vi "bigmcs.vi"(5 "Spinal Column Out":T2={"Red MOT 88 Inputs"={"Active Device"="", "Active Channels"=[], "Waveform Parameters"=[], "Active Phases"=[], "Phase Times"=[], "Trigger Channel"=""}, "6713 Blue MOT"={"Active Device"="", "Active Channels"=[], "Waveform Parameters"=[], "Active Phases"=[], "Phase Times"=[], "Trigger Channel"="", "FIFO Buffer Size"=0.0}, "Instructions"=[], "Red MOT 87 Inputs"={"Active Device"="", "Active Channels"=[], "Waveform Parameters"=[], "Active Phases"=[], "Phase Times"=[], "Trigger Channel"=""}, "ODT Params"={"Waveform Parameters"=[], "Active Phases"=[], "Active Channels"=[], "Phase Times (s)"=[], "Active Device"="", "Trigger Channel"="", "Evaporation Phase"=0.0, "Evaporation Channel"=0.0}, "Agilent E3631A Settings"={"VISA resource name"="", "Voltage Set (6V max)"=0.0, "Current Set (5A max)"=0.0, "Voltage Set (25V max)"=0.0, "Current Set (1A max)"=0.0}, "PixelFly Initialization"={"Exposure mode"=0, "exp time"=0, "exp level"=0, "gain"=0, "boardid in"=0, "offset"=0, "V bin"=0, "H bin"=0, "trigger"=FALSE, "Bit depth"=0}, "Scan Parameters"={"Initial Values"=[], "Final Values"=[], "Step Sizes"=[], "Parameters to Change"=[], "Channels to Change"=[], "Number of Parameters to Scan"=0, "Parameter Nickname (no spaces)"=[], "Scan Base Name"="", "Raw_Data Folder"=path "", "ROI Parameters"={"Background Radius"=0.0, "Atom Radius"=0.0, "X Center"=0.0, "Y Center"=0.0}, "Drop Time (ms)"=0.0, "ODT VCA 1 Channel"=0.0, "ODT VCA 2 Channel"=0.0, "Phases To Change"=[], "Scan Pulseblaster Channel With Parameter"={"Change PB Time Toggle"=FALSE, "PB Channel"=0.0, "Parameter Number"=0.0}, "Preserve Waveform\nContinuity"=FALSE, "Generated Array Type"=enum."Custom Array From File", "Principle Quantum #"=0, "Angular Momentum"=enum."s", "Ramp Delay Channel"=0, "ODT Hold Channel"=0, "MCS ROI Min"=0, "MCS ROI Max"=0, "Master Batch Fourth Column"=0.0}, "MCS Parameters"={"Scan Length (Bins)"=0.0, "Dwell Time (s)"=0.0, "Gate Channel Settings"={"Threshold (V)"=0.0, "Edge"=enum."Falling", "Input Impedence"=enum."1k Ohm"}, "Trig Channel Settings"={"Threshold (V)"=0.0, "Edge"=enum."Falling", "Input Impedence"=enum."1k Ohm"}, "Input 1 Settings"={"Threshold (V)"=0.0, "Edge"=enum."Falling", "Input Impedence"=enum."1k Ohm"}, "Input 2 Settings"={"Threshold (V)"=0.0, "Edge"=enum."Falling", "Input Impedence"=enum."1k Ohm"}, "Number of Sweeps"=0, "Number of Sequential Cycles"=0.0, "Number of Sequences"=0.0, "Sweep Preset"=FALSE, "Sequential Mode"=FALSE, "DAC 1 Ramp Settings"={"Ramp Mode"=enum."Fixed", "Ramp Start Value (V)"=0.0, "Ramp Length (Steps)"=0, "Step Width (bins)"=0, "Step Size (V)"=0.0}, "DAC 2 Output (V)"=0.0, "SYNC Output"=enum."40 MHz Clock", "ROI Min"=0, "ROI Max"=0, "Dual MCS Mode"=FALSE, "DAC 2 Toggle"=FALSE, "MCS on/off"=FALSE, "ROI Max 2"=1, "ROI Min 2"=0, "Sum ROI Only"=FALSE, "Use ROI For \nEach Loop"=FALSE}, "PicoScope"={"Channel A Settings"={"Enabled"=FALSE, "Coupling"=0, "Range"=0, "Analogue Offset"=0.0}, "Channel B Settings"={"Enabled"=FALSE, "Coupling"=0, "Range"=0, "Analogue Offset"=0.0}, "Trigger Options"={"Trigger Enabled"=FALSE, "Trigger Source"=enum."Channel A", "Trigger Threshold (-5 to 5 V)"=0.0, "Trigger Slope"=0, "Trigger Delay (ms)"=0.0, "Auto Trigger Time (ms)"=0}, "Pico Scope Inititalization Settings"={"USB Power"=FALSE, "Use Serial Number"=FALSE, "Resolution"=0, "Serial Number"="", "Handle"=0}, "Use PicoScope?"=FALSE, "Acquisition Settings"={"Pre Trigger Time (s)"=0.0, "Post Trigger Time (s)"=0.0, "Resolution (s)"=0.0, "Four Channel Device"=FALSE, "Number of Captures"=0.0}}, "Ramp Delay Settings"={"Insert Delays"=FALSE, "Number of loops"=0, "Insert after instruction"=0, "Random"=FALSE, "Initial Delay Time (s)"=0.0, "Final Delay Time (s)"=0.0, "Delay Step (s)"=0.0, "Delay Column"=0.0, "Loop Hold Column"=0.0, "Field Ramp Column"=0.0, "Excitation Column"=0.0, "Hold + Delay + Excitation Time"=0.0, "Ascending/Descending"=FALSE, "Subroutine A"=[]}, "6229 Green Lattice Inputs"={"Active Device"="", "Active Channels"=[], "Waveform Parameters"=[], "Active Phases"=[], "Phase Times"=[], "Trigger Channel"="", "FIFO Buffer Size"=0.0}, "Synth Controls 1"={"Channel Settings"=[], "Active Channels"=[], "COM Port"="", "Table Mode"={"Table Mode On/Off"=FALSE, "Initial Frequency (MHz)"=0.0, "FinalFreq"=0.0, "Frequency Step (MHz)"=0.0, "Ascending/Descending"=FALSE, "Random"=FALSE}}, "Synth Controls 2"={"Channel Settings"=[], "Active Channels"=[], "COM Port"="", "Table Mode"={"Table Mode On/Off"=FALSE, "Initial Frequency (MHz)"=0.0, "FinalFreq"=0.0, "Frequency Step (MHz)"=0.0, "Ascending/Descending"=FALSE, "Random"=FALSE}}, "Indicator References"={"Blue MOT Waveform Graph"=refnum, "Red 88 Waveform Graph"=refnum, "Red 87 Waveform Graph"=refnum, "ODT Waveform Graph"=refnum, "Green Lattice Waveform Graph"=refnum, "Agilent E3631A Measurements"=refnum}} {"Red MOT 88 Inputs"."Phase Times" format="%.0p"; "Red MOT 88 Inputs"."Waveform Parameters"."Degree" min=1; "6713 Blue MOT"."Phase Times" format="%.3f"; "Instructions"."Time (s)" min=5e-08 format="%.2p"; "Instructions"."Op Code" items=["Continue", "Stop", "Loop", "End Loop", "JSR", "RTS", "Go To", "Long Delay", "Wait"]; "Instructions"."Instruct Data" format="%#.2p"; "Red MOT 87 Inputs"."Phase Times" format="%.0p"; "Red MOT 87 Inputs"."Waveform Parameters"."Degree" min=1; "ODT Params"."Evaporation Channel" min=0.0 max=1.0 step=1.0; "ODT Params"."Evaporation Phase" min=0.0 max=4.0 step=1.0; "ODT Params"."Phase Times (s)" format="%#_6p"; "Agilent E3631A Settings"."Current Set (1A max)" format="%.3g"; "Agilent E3631A Settings"."Voltage Set (25V max)" format="%.3g"; "Agilent E3631A Settings"."Current Set (5A max)" format="%.3g"; "Agilent E3631A Settings"."Voltage Set (6V max)" format="%.3g"; "PixelFly Initialization"."Bit depth" items=["2"=1]; "PixelFly Initialization"."H bin" items=["1", "2"]; "PixelFly Initialization"."V bin" items=["1", "2"]; "PixelFly Initialization"."boardid in" min=0 max=3 step=1; "PixelFly Initialization"."gain" items=["Low (X1)", "High (X2)"]; "PixelFly Initialization"."exp level" min=0 max=255 step=1; "PixelFly Initialization"."exp time" min=1 max=10000; "PixelFly Initialization"."Exposure mode" items=["Asynch shutter", "Double shot", "Video mode", "Auto exposure"]; "Scan Parameters"."Drop Time (ms)" min=1.0; "Scan Parameters"."Number of Parameters to Scan" min=1; "MCS Parameters"."ROI Max 2" min=1; "MCS Parameters"."ROI Min 2" min=0; "MCS Parameters"."ROI Max" min=1; "MCS Parameters"."ROI Min" min=0; "MCS Parameters"."DAC 2 Output (V)" min=-10.0 max=10.0 step=0.00488; "MCS Parameters"."DAC 1 Ramp Settings"."Step Size (V)" min=0.0 max=10.0 step=0.00244 format="%#_4g"; "MCS Parameters"."DAC 1 Ramp Settings"."Step Width (bins)" min=1; "MCS Parameters"."DAC 1 Ramp Settings"."Ramp Length (Steps)" min=1; "MCS Parameters"."DAC 1 Ramp Settings"."Ramp Start Value (V)" min=0.0 max=10.0 step=0.00244; "MCS Parameters"."Number of Sweeps" min=0 format="%.0p"; "MCS Parameters"."Input 2 Settings"."Threshold (V)" min=-2.5 max=2.5 step=0.001; "MCS Parameters"."Input 1 Settings"."Threshold (V)" min=-2.5 max=2.5 step=0.001; "MCS Parameters"."Trig Channel Settings"."Threshold (V)" min=-2.5 max=2.5 step=0.001; "MCS Parameters"."Gate Channel Settings"."Threshold (V)" min=-2.5 max=2.5 step=0.001; "MCS Parameters"."Dwell Time (s)" min=1e-07 step=2.5e-08 format="%#_6p"; "MCS Parameters"."Scan Length (Bins)" min=64.0 max=524288.0 format="%#_7f"; "PicoScope"."Acquisition Settings"."Resolution (s)" min=8e-09 max=34.36 step=8e-09 format="%#_6p"; "PicoScope"."Acquisition Settings"."Post Trigger Time (s)" min=0.0 format="%#_6p"; "PicoScope"."Acquisition Settings"."Pre Trigger Time (s)" min=0.0 format="%#_6p"; "PicoScope"."Pico Scope Inititalization Settings"."Resolution" items=["8-bit", "12-bit", "14-bit", "15-bit (max. 2 ch.)", "16-bit (max. 1 ch.)"]; "PicoScope"."Trigger Options"."Trigger Slope" items=["Rising"=2, "Falling"=3]; "PicoScope"."Channel B Settings"."Range" items=["10 mV", "20 mV", "50 mV", "100 mV", "200 mV", "500 mV", "1 V", "2 V", "5 V", "10 V", "20 V", "50 V ", "100 V"]; "PicoScope"."Channel B Settings"."Coupling" items=["AC", "DC"]; "PicoScope"."Channel A Settings"."Range" items=["10 mV", "20 mV", "50 mV", "100 mV", "200 mV", "500 mV", "1 V", "2 V", "5 V", "10 V", "20 V", "50 V ", "100 V"]; "PicoScope"."Channel A Settings"."Coupling" items=["AC", "DC"]; "Ramp Delay Settings"."Subroutine A"."Time (s)" min=5e-08 format="%.2p"; "Ramp Delay Settings"."Subroutine A"."Op Code" items=["Continue", "Stop", "Loop", "End Loop", "JSR", "RTS", "Go To", "Long Delay", "Wait"]; "Ramp Delay Settings"."Subroutine A"."Instruct Data" format="%#.2p"; "Ramp Delay Settings"."Insert after instruction" min=0; "Ramp Delay Settings"."Delay Step (s)" min=5e-08 format="%#_6p"; "Ramp Delay Settings"."Final Delay Time (s)" min=5e-08 format="%#_6p"; "Ramp Delay Settings"."Initial Delay Time (s)" min=5e-08 format="%#_6p"; "6229 Green Lattice Inputs"."Phase Times" format="%.3f"; "6229 Green Lattice Inputs"."Waveform Parameters"."Degree" min=1}, 7 "Synth Freq":dbl, 8 "MCS Counts Out":u32[][](graph)=[[0, 0, 0, 0, 0, 0, 0, 0, 0, 0, 0, 0, 0, 0, 0, 0, 0, 0, 0, 0, 0, 0, 0, 0, 0, 0, 0, 0, 0, 0, 0, 0, 0, 0, 0, 0, 0, 0, 0, 0, 0, 0, 0, 0, 0, 0, 0, 0, 0, 0, 0, 0, 0, 0, 0, 0, 0, 0, 0, 0, 0, 0, 0, 0, 0, 0, 0, 0, 0, 0, 0, 0, 0, 1, 1, 0, 0, 0, 0, 0, 2, 0, 0, 0, 0, 0, 0, 0, 0, 0, 0, 0, 0, 1, 3, 1, 0, 0, 0, 0, 0, 0, 0, 0, 0, 0, 0, 0, 0, 0, 0, 0, 0, 0, 0, 0, 0, 0, 0, 0, 0, 0, 0, 0, 0, 0, 0, 0, 0, 0, 0, 0, 0, 0, 0, 0, 0, 0, 0, 0, 0, 0, 0, 0, 0, 0, 0, 0, 0, 0, 0, 0, 0, 0, 0, 0, 0, 0, 0, 0, 0, 0, 0, 0, 0, 0, 0, 0, 0, 0, 0, 0, 0, 0, 1, 0, 0, 0, 0, 0, 0, 0, 0, 0, 0, 0, 0, 0, 0, 0, 0, 0, 0, 0, 0, 0, 0, 0, 0, 0, 0, 0, 0, 0, 0, 0, 0, 0, 0, 0, 0, 0, 0, 0, 0, 0, 0, 0, 0, 0, 0, 0, 0, 0, 0, 0, 0, 0, 0, 0, 0, 0, 0, 0, 0, 0, 0, 0, 0, 0, 0, 0, 0, 0, 0, 0, 0, 0, 0, 0]], 9 "Tau Array":dbl[](array[numeric]), 10 "Sum #":dbl, 11 "Sum in":u32[][](graph)) -> ()   [LabVIEW 2015]
uses:
  Controls/Spinal Column/spinal_column.ctl
  6733_Red_MOT/6733_control_panel.ctl
  6733_Red_MOT/6733_waveform_parameter_array.ctl
  6733_Red_MOT/6733_waveform_item.ctl
  6733_Red_MOT/Neutral_voltage_conversion_control.ctl
  Controls/6713/6713_waveform_generation.ctl
  Controls/6713/6713_waveform_parameter_array.ctl
  Controls/6713/6713_static_waveform_item.ctl
  Controls/PulseBlaster/Instructions_Cluster.ctl
  Neutral_DAQ/6221 arb waveforms/6221_panel.ctl
  Neutral_DAQ/6221 arb waveforms/6221_waveform_param.ctl
  Controls/Agilent E3631A/Settings_Control.ctl
  Controls/PixelFly/Camera_Initialization.ctl
  Controls/ScanParameters/ScanParametersPanel.ctl
  Controls/ScanParameters/ParameterToChange.ctl
  Controls/ScanParameters/ROI_set.ctl
  Controls/ScanParameters/ScanPBandParam.ctl
  Controls/MCS/mcs_control_panel.ctl
  Controls/MCS/mcs_channel.ctl
  Controls/MCS/ramp_control.ctl
  Controls/PicoScope/pico_control_panel.ctl
  Controls/PicoScope/pico_channel_settings.ctl
  Controls/PicoScope/pico_trigger.ctl
  Controls/PicoScope/pico_init_settings.ctl
  Controls/PulseBlaster/delay_control_3..ctl
  Controls/6229/6229_arb_waveform_generation.ctl
  Controls/Synth_409b/Synth_controls.ctl
  Controls/Synth_409b/synth_channel.ctl
  Controls/Synth_409b/table_mode.ctl
  <vilib>/Utility/file.llb/Write To Spreadsheet File (DBL).vi
  <vilib>/Analysis/NI_AALPro.lvlib
panel:
  in  "Trace Scale":bool caption="Linear / Logrithmic"
  in  "Sum Scale":bool caption="Linear / Logrithmic"
  in  "Record Lifetime":bool
  in  "file path (dialog if empty)":path
  out "Lifetime Running Average":dbl[][](graph)
  out "Sum graph":u32[][](graph)
  out "error out":errorcluster
  out "XY Graph 3":cluster{"Tau Array":dbl[], u32[]}[](graph)
  out "Lifetimes":dbl[][](graph)
  out "Lifetimes":dbl[](array[numeric])
  in  "parameter bounds":T1={"amp min"=-inf, "amp max"=inf, "damping min"=-inf, "damping max"=inf, "offset min"=0.0, "offset max"=0.0}
  in  "Clear Graph":bool
  out "appended array":cluster{"Sum #":dbl, "Synth Freq":dbl}[](array[cluster])
  out "XY Graph":cluster{"X":dbl, "Y":dbl}[](graph)
  # "Channel 0"
  # "Channel 1"
  # "Channel 2"
  # "Channel 3"
  # "Channel 4"
  # "Channel 5"
  # "Channel 7"
  # "Channel 7"
  # "(0) 689 Center Freq"
  # "(1) 689 Dither Amp"
  # "(2) 689 Power Lock"
  # "(3) Red MOT Field Grad"
  # "Channel 0"
  # "Channel 1"
  # "Channel 2"
  # "Channel 3"
  # "Channel 4"
  # "Channel 5"
  # "Channel 7"
  # "Channel 7"
  # "6V Output Settings"
  # "25V Output Settings"
  # "Select a PB Channel to set with a phase time\nfor evaporation or whatever"
  # "(0) Arm A"
  # "(1) Arm B"
  # "(2) Arm C"
  # "(3) Unused"
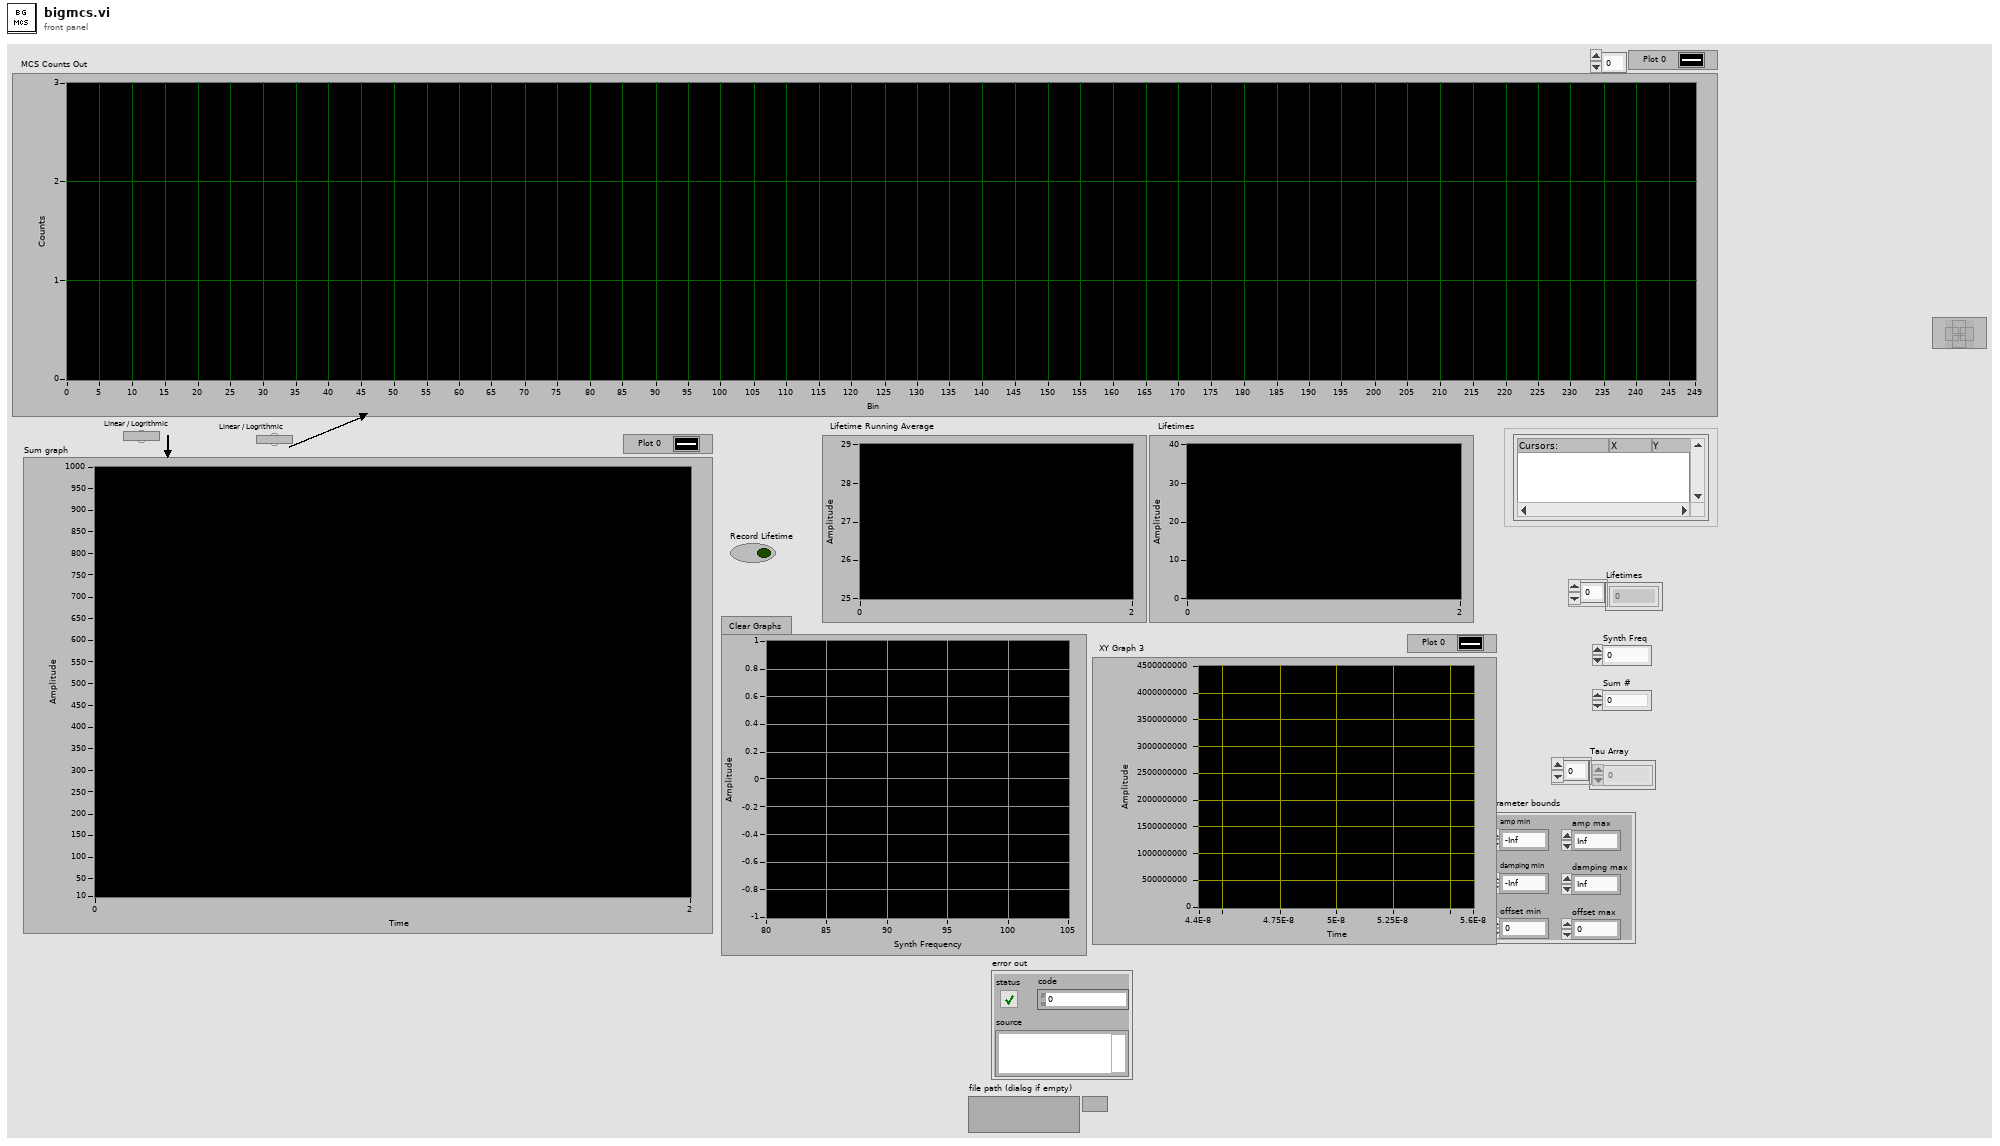
[diagram p1: front panel]
types:
  T1 = cluster{"amp min":dbl, "amp max":dbl, "damping min":dbl, "damping max":dbl, "offset min":dbl, "offset max":dbl}
  T2 = typedef "spinal_column.ctl" = cluster{"Red MOT 88 Inputs":T3, "6713 Blue MOT":T7, "Instructions":T10, "Red MOT 87 Inputs":T3, "ODT Params":T11, "Agilent E3631A Settings":T13, "PixelFly Initialization":T14, "Scan Parameters":T15, "MCS Parameters":T19, "PicoScope":T22, "Ramp Delay Settings":T26, "6229 Green Lattice Inputs":T27, "Synth Controls 1":T28, "Synth Controls 2":T28, "Indicator References":cluster{"Blue MOT Waveform Graph":refnum<vi>, "Red 88 Waveform Graph":refnum<vi>, "Red 87 Waveform Graph":refnum<vi>, "ODT Waveform Graph":refnum<vi>, "Green Lattice Waveform Graph":refnum<vi>, "Agilent E3631A Measurements":refnum<vi>}}
  T3 = typedef "6733_control_panel.ctl" = cluster{"Active Device":string, "Active Channels":bool[], "Waveform Parameters":T4, "Active Phases":bool[], "Phase Times":dbl[], "Trigger Channel":tag}
  T4 = typedef "6733_waveform_parameter_array.ctl" = T5[][]
  T5 = typedef "6733_waveform_item.ctl" = cluster{"Function":enum16{"Polynomial", "Exponential", "Constant"}, "Initial":dbl, "Final":dbl, "Degree":i8, "Nickname":string, "Conversion":T6, "Constant":dbl}
  T6 = typedef "Neutral_voltage_conversion_control.ctl" = enum16{"Volts", "B Field Grad (G/cm)", "Red MOT Center Freq (MHz)", "Red Dither Pk(kHz)", "Red Power (mW)", "ODT Sheet Trap Power (W)", "ODT Loading Trap Power (W)"}
  T7 = typedef "6713_waveform_generation.ctl" = cluster{"Active Device":string, "Active Channels":bool[], "Waveform Parameters":T8, "Active Phases":bool[], "Phase Times":dbl[], "Trigger Channel":tag, "FIFO Buffer Size":dbl}
  T8 = typedef "6713_waveform_parameter_array.ctl" = T9[][]
  T9 = typedef "6713_static_waveform_item.ctl" = cluster{"Constant":dbl, "Nickname":string, "Conversion":T6}
  T10 = typedef "Instructions_Cluster.ctl" = cluster{"Instruct Data":i32, "Op Code":i32, "Flags":bool[], "Comments":string, "Time (s)":dbl, "Column Number":string, "Array":string[]}[]
  T11 = typedef "6221_panel.ctl" = cluster{"Waveform Parameters":T12[][], "Active Phases":bool[], "Active Channels":bool[], "Phase Times (s)":dbl[], "Active Device":string, "Trigger Channel":tag, "Evaporation Phase":dbl, "Evaporation Channel":dbl}
  T12 = typedef "6221_waveform_param.ctl" = cluster{"Initial Value":dbl, "Final Value":dbl, "Tau":dbl, "Eta":dbl, "Nickname":string, "Enum":enum16{"Volts to Volts", "Power Law", "Evaporation Formula"}, "Conversion":T6}
  T13 = typedef "Settings_Control.ctl" = cluster{"VISA resource name":refnum<visa-resource-name>, "Voltage Set (6V max)":dbl, "Current Set (5A max)":dbl, "Voltage Set (25V max)":dbl, "Current Set (1A max)":dbl}
  T14 = typedef "Camera_Initialization.ctl" = cluster{"Exposure mode":u16, "exp time":i32, "exp level":i32, "gain":i32, "boardid in":i32, "offset":i32, "V bin":i32, "H bin":i32, "trigger":bool, "Bit depth":i32}
  T15 = typedef "ScanParametersPanel.ctl" = cluster{"Initial Values":dbl[], "Final Values":dbl[], "Step Sizes":dbl[], "Parameters to Change":T16[], "Channels to Change":dbl[], "Number of Parameters to Scan":i32, "Parameter Nickname (no spaces)":string[], "Scan Base Name":string, "Raw_Data Folder":path, "ROI Parameters":T17, "Drop Time (ms)":dbl, "ODT VCA 1 Channel":dbl, "ODT VCA 2 Channel":dbl, "Phases To Change":dbl[], "Scan Pulseblaster Channel With Parameter":T18, "Preserve Waveform\nContinuity":bool, "Generated Array Type":enum16{"Custom Array From File", "Default (old way)"}, "Principle Quantum #":i32, "Angular Momentum":enum16{"s", "p", "d", "f", "g", "h"}, "Ramp Delay Channel":i32, "ODT Hold Channel":i32, "MCS ROI Min":i32, "MCS ROI Max":i32, "Master Batch Fourth Column":dbl}
  T16 = typedef "ParameterToChange.ctl" = enum16{"Delay single delay time", "Dummy Variable", "Delay Exposure", "PB Loops", "Number of Delay Loops", "Subroutine A Time", "Subroutine B Time", "Synth Amplitude", "Synth Frequency", "Synth Phase", "ODT Params Phase Time", "ODT Params Tau", "ODT Params Final Voltage", "ODT Params Initial Voltage", "ODT Params Eta", "Red Mot 88 Phase Time", "Red Mot 87 Phase Time", "Red Mot 88 Final Voltage", "Red Mot 88 Initial Voltage", "Red Mot 87 Final Voltage", "Red Mot 87 Initial Voltage", "PulseBlaster", "6713 Voltage"}
  T17 = typedef "ROI_set.ctl" = cluster{"Background Radius":dbl, "Atom Radius":dbl, "X Center":dbl, "Y Center":dbl}
  T18 = typedef "ScanPBandParam.ctl" = cluster{"Change PB Time Toggle":bool, "PB Channel":dbl, "Parameter Number":dbl}
  T19 = typedef "mcs_control_panel.ctl" = cluster{"Scan Length (Bins)":dbl, "Dwell Time (s)":dbl, "Gate Channel Settings":T20, "Trig Channel Settings":T20, "Input 1 Settings":T20, "Input 2 Settings":T20, "Number of Sweeps":i32, "Number of Sequential Cycles":dbl, "Number of Sequences":dbl, "Sweep Preset":bool, "Sequential Mode":bool, "DAC 1 Ramp Settings":T21, "DAC 2 Output (V)":dbl, "SYNC Output":enum16{"40 MHz Clock", "Gate Disc Signal", "Trigger Disc Signal", "Counter 1 Disc Signal", "Counter 2 Disc Signal", "Definitely Not Used", "Not Used", "1 kHz Signal", "Also Not Used", "MCS On/Off", "End of Time Bin", "Ramp Increment Trig", "Step Count Trigger", "'GO'-Line", "Ramp Down Trigger", "Logic 1"}, "ROI Min":i32, "ROI Max":i32, "Dual MCS Mode":bool, "DAC 2 Toggle":bool, "MCS on/off":bool, "ROI Max 2":i32, "ROI Min 2":i32, "Sum ROI Only":bool, "Use ROI For \nEach Loop":bool}
  T20 = typedef "mcs_channel.ctl" = cluster{"Threshold (V)":dbl, "Edge":enum16{"Falling", "Rising"}, "Input Impedence":enum16{"1k Ohm", "50 Ohm"}}
  T21 = typedef "ramp_control.ctl" = cluster{"Ramp Mode":enum16{"Fixed", "Triangle", "Sawtooth"}, "Ramp Start Value (V)":dbl, "Ramp Length (Steps)":i32, "Step Width (bins)":i32, "Step Size (V)":dbl}
  T22 = typedef "pico_control_panel.ctl" = cluster{"Channel A Settings":T23, "Channel B Settings":T23, "Trigger Options":T24, "Pico Scope Inititalization Settings":T25, "Use PicoScope?":bool, "Acquisition Settings":cluster{"Pre Trigger Time (s)":dbl, "Post Trigger Time (s)":dbl, "Resolution (s)":dbl, "Four Channel Device":bool, "Number of Captures":dbl}}
  T23 = typedef "pico_channel_settings.ctl" = cluster{"Enabled":bool, "Coupling":i16, "Range":u16, "Analogue Offset":sgl}
  T24 = typedef "pico_trigger.ctl" = cluster{"Trigger Enabled":bool, "Trigger Source":enum16{"Channel A", "Channel B", "Channel C", "Channel D", "Ext."}, "Trigger Threshold (-5 to 5 V)":dbl, "Trigger Slope":u16, "Trigger Delay (ms)":dbl, "Auto Trigger Time (ms)":i16}
  T25 = typedef "pico_init_settings.ctl" = cluster{"USB Power":bool, "Use Serial Number":bool, "Resolution":i32, "Serial Number":string, "Handle":i16}
  T26 = typedef "delay_control_3..ctl" = cluster{"Insert Delays":bool, "Number of loops":i32, "Insert after instruction":i32, "Random":bool, "Initial Delay Time (s)":dbl, "Final Delay Time (s)":dbl, "Delay Step (s)":dbl, "Delay Column":dbl, "Loop Hold Column":dbl, "Field Ramp Column":dbl, "Excitation Column":dbl, "Hold + Delay + Excitation Time":dbl, "Ascending/Descending":bool, "Subroutine A":T10}
  T27 = typedef "6229_arb_waveform_generation.ctl" = cluster{"Active Device":string, "Active Channels":bool[], "Waveform Parameters":T4, "Active Phases":bool[], "Phase Times":dbl[], "Trigger Channel":tag, "FIFO Buffer Size":dbl}
  T28 = typedef "Synth_controls.ctl" = cluster{"Channel Settings":T29[], "Active Channels":bool[], "COM Port":refnum<visa-resource-name>, "Table Mode":T30}
  T29 = typedef "synth_channel.ctl" = cluster{"Voltage (Amp.) ":dbl, "Frequency (MHz)":dbl, "Phase (deg)":dbl, "Nickname":string}
  T30 = typedef "table_mode.ctl" = cluster{"Table Mode On/Off":bool, "Initial Frequency (MHz)":dbl, "FinalFreq":dbl, "Frequency Step (MHz)":dbl, "Ascending/Descending":bool, "Random":bool}
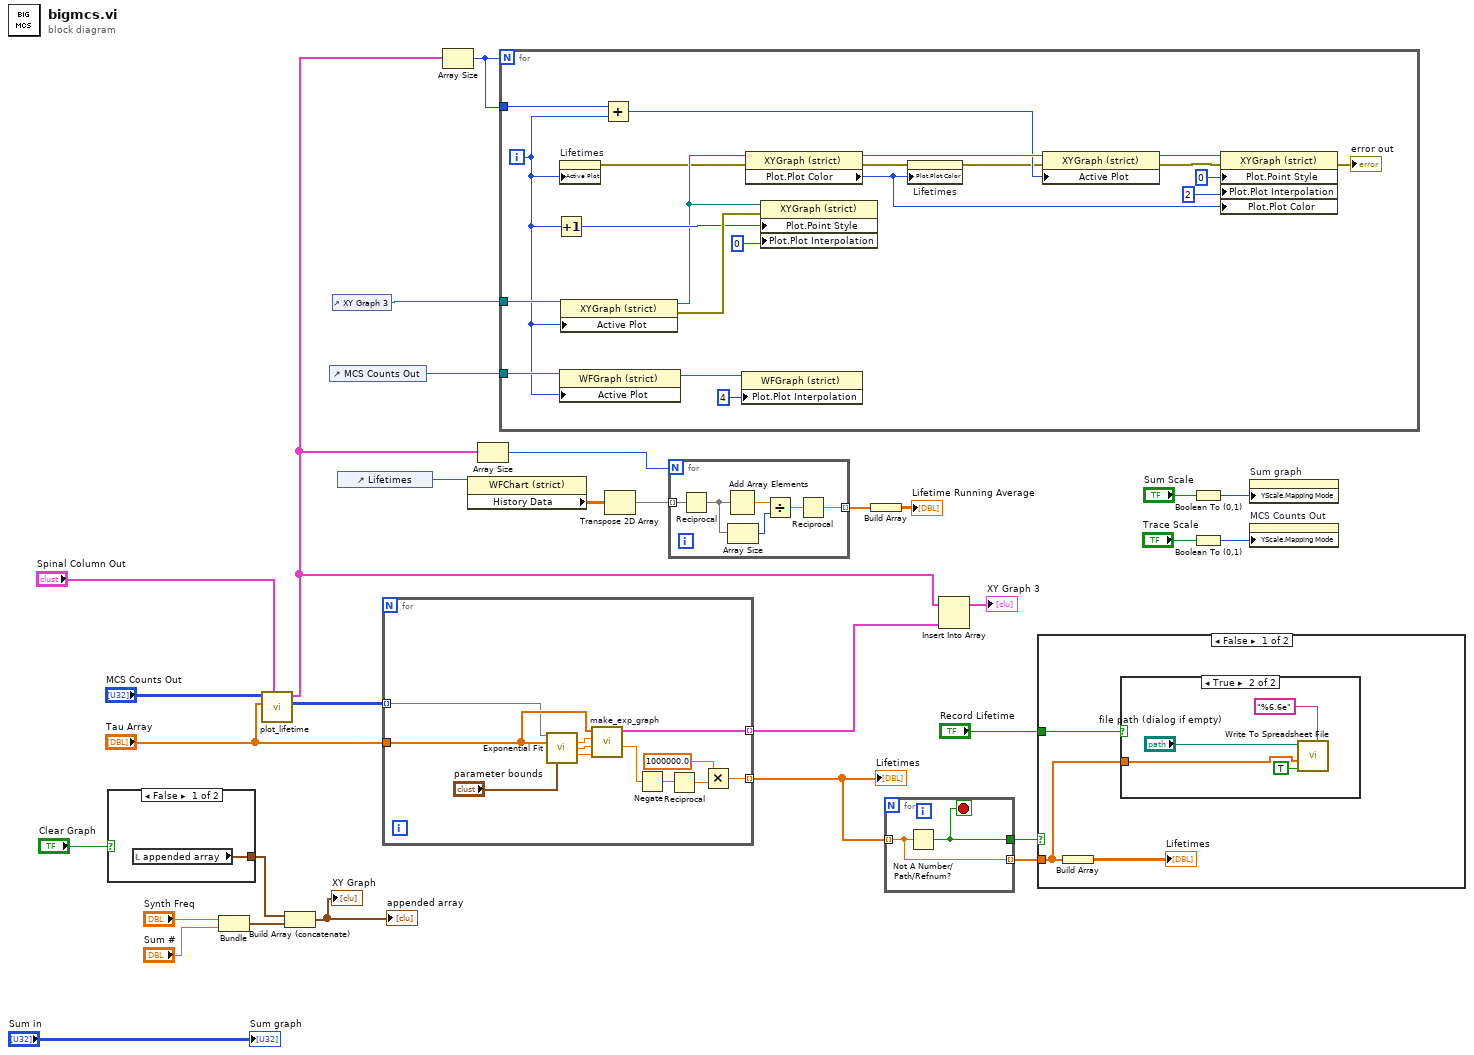
[diagram p0: block diagram]
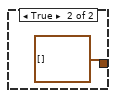
[diagram p4: hidden frame]
diagram:
  n1 = case shown="False" "Clear Graph" {
    tunnel: [w32 cluster{"Sum #":dbl, "Synth Freq":dbl}[] [] ("appended array")] -> w29
    frame False {
      n2 = local read "appended array"() -> (w32:cluster{"Sum #":dbl, "Synth Freq":dbl}[])
    }
    frame True {
    }
  }
  n3 = Bundle("Synth Freq"="Synth Freq", "Sum #"="Sum #") -> (w31:cluster{"Synth Freq":dbl, "Sum #":dbl})  [unwired: 1 in]
  n4 = call "plot_lifetime.vi"("Spinal Column Out"="Spinal Column Out", "Tau Array"="Tau Array", "MCS Counts Out"="MCS Counts Out") -> ("Array"=w23:u32[][], "XY Graph"=w10:cluster{"Tau Array":dbl[], u32[]}[])  [unwired: 7 in]
  n5 = Build Array (concatenate)(w29, w31) -> (→"XY Graph" →"appended array":cluster{"Synth Freq":dbl, "Sum #":dbl}[])
  n6 = control-ref of="MCS Counts Out"() -> (w16:refnum<vi>)
  n7 = control-ref of="XY Graph 3"() -> (w20:refnum<vi>)
  n8 = control-ref of="Lifetimes"() -> (w15:refnum<vi>)
  n9 = for {
    tunnel: "Tau Array" -> [w40]
    tunnel: [w41] -> w8 mode=indexing
    tunnel: [w35] -> w22 mode=indexing
    tunnel: w23 -> [w34] mode=indexing
    n10 = call <vilib>:"Exponential Fit.vi"("Y"=w34, "X"=w40, "parameter bounds"="parameter bounds") -> ("amplitude"=w39:dbl, "damping"=w38:dbl, "offset"=w37:dbl)  [unwired: 7 in, 3 out]
    n11 = call "make_exp_graph.vi"("Offset"=w37, "Damping"=w38, "Amplitude"=w39, "Tau Array In"=w40) -> ("Damping Out"=w36:dbl, "output cluster"=w35:cluster{dbl[], dbl[]})  [unwired: 4 in, 2 out]
    n12 = Negate(x=w36) -> (-x=w44:dbl)
    n13 = Reciprocal(x=w44) -> (1/x=w43:dbl)
    n14 = Multiply(x=1000000.0, y=w43) -> (x*y=w41:dbl)
  }
  "Lifetimes" <- w8
  n15 = Array Size(array=w10) -> (size(s)=w19:i32)
  n16 = property class="WFChart (strict)"(reference=w15) -> ("History Data"=w11:dbl[][])  [unwired: 1 in, 2 out]
  n17 = Array Size(array=w10) -> (size(s)=w9:i32)
  n18 = for {
    N: w19 -> [_]
    tunnel: w20 -> [w63]
    tunnel: w19 -> [w59]
    tunnel: w16 -> [w49]
    i -> [w46]
    n19 = Increment(x=w46) -> (x+1=w64:i32)
    n20 = property on="Lifetimes" class="WFChart (strict)"("Active Plot"=w46) -> (error out=w61:errorcluster)  [unwired: 2 in, 1 out]
    n21 = property class="WFGraph (strict)"(reference=w49, "Active Plot"=w46) -> (reference out=w48:refnum<vi>)  [unwired: 1 in, 1 out]
    n22 = property on="Property Node" class="XYGraph (strict)"(reference=w63, "Active Plot"=w46) -> (reference out=w62:refnum<vi>, error out=w66:errorcluster)  [unwired: 1 in]
    n23 = Add(x=w59, y=w46) -> (x+y=w57:i32)
    n24 = property class="WFGraph (strict)"(reference=w48, "Plot.Plot Interpolation"=u8 4) -> ()  [unwired: 1 in, 2 out]
    n25 = property on="Property Node" class="XYGraph (strict)"(reference=w62, error in=w61) -> (reference out=w58:refnum<vi>, error out=w60:errorcluster, "Plot.Plot Color"=w53:u32)
    n26 = property on="Property Node" class="XYGraph (strict)"(reference=w62, error in=w66, "Plot.Point Style"=w64, "Plot.Plot Interpolation"=u8 0 ("Plot.Line Style")) -> ()  [unwired: 2 out]
    n27 = property on="Lifetimes" class="WFChart (strict)"(error in=w60, "Plot.Plot Color"=w53) -> (error out=w56:errorcluster)  [unwired: 1 in, 1 out]
    n28 = property on="Property Node" class="XYGraph (strict)"(reference=w58, error in=w56, "Active Plot"=w57) -> (reference out=w55:refnum<vi>, error out=w51:errorcluster)
    n29 = property on="Property Node" class="XYGraph (strict)"(reference=w55, error in=w51, "Plot.Point Style"=u8 0, "Plot.Plot Interpolation"=u8 2, "Plot.Plot Color"=w53) -> (error out=→"error out":errorcluster)  [unwired: 1 out]
  }
  n30 = Transpose 2D Array(2D array=w11) -> (transposed array=w12:dbl[][])
  n31 = for {
    N: w9 -> [_]
    tunnel: w12 -> [w70] mode=indexing
    tunnel: [w67] -> w14 mode=indexing
    n32 = Reciprocal(x=w70) -> (1/x=w69:dbl[])
    n33 = Add Array Elements(numeric array=w69) -> (sum=w72:dbl)
    n34 = Array Size(array=w69) -> (size(s)=w71:i32)
    n35 = Divide(x=w72, y=w71) -> (x/y=w68:dbl)
    n36 = Reciprocal(x=w68) -> (1/x=w67:dbl)
  }
  n37 = Build Array(w14) -> (→"Lifetime Running Average":dbl[][])
  n38 = for {
    tunnel: w8 -> [w73] mode=indexing
    tunnel: [w74] -> w7
    tunnel: [w73] -> w6 mode=indexing
    stop <- w74 stop-if-true
    n39 = Not A Number/Path/Refnum?(number/path/refnum=w73) -> (NaN/Path/Refnum?=w74:bool)
  }
  n40 = Insert Into Array(array=w10, new element=w22) -> (→"XY Graph 3":cluster{"Tau Array":dbl[], u32[]}[])  [unwired: 1 in]
  n41 = case shown="False" w7 {
    tunnel: w6 -> [w76 _]
    tunnel: "Record Lifetime" -> [w75 _]
    frame False {
      n42 = Build Array(w76) -> (→"Lifetimes":dbl[][])
      n43 = case shown="True" w75 {
        tunnel: w76 -> [_ w81]
        frame False {
        }
        frame True {
          n44 = call-poly <vilib>:"Write To Spreadsheet File.vi"("format (%.3f)"="%6.6e", "append to file? (new file:F)"=TRUE, "1D data"=w81, "file path (dialog if empty)"="file path (dialog if empty)") -> ()  [unwired: 4 in, 1 out]
        }
      }
    }
    frame True {
    }
  }
  n45 = Boolean To (0,1)(Boolean="Sum Scale") -> (0, 1=w2:i16)
  n46 = Boolean To (0,1)(Boolean="Trace Scale") -> (0, 1=w1:i16)
  n47 = property on="Sum graph" class="WFChart (strict)"("YScale.Mapping Mode"=w2) -> ()  [unwired: 2 in, 2 out]
  n48 = property on="MCS Counts Out" class="WFGraph (strict)"("YScale.Mapping Mode"=w1) -> ()  [unwired: 2 in, 2 out]
  "Sum graph" <- "Sum in"
